vi "Calc Type.vi"(11 "Div Calc in":refnum<class "Div Calc.lvclass">) -> (2 "Calc Type":string)   [LabVIEW 2020, in "VolatusCalcs.lvlib" / "Div Calc.lvclass"]
uses:
  Div Calc.lvclass
  Div Calc.lvclass/Div Calc.ctl
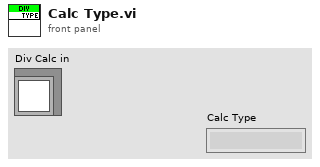
[diagram p1: front panel]
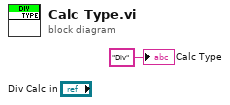
[diagram p0: block diagram]
diagram:
  "Calc Type" <- "Div" ("Calc Type")
